vi "LLB - Header.vi"(7 "Msg Chain":string, 8 "error in (no error)":errorcluster {"code" format="Error %.0f"}, 10 "LLBs":refnum<class "LLB Documentation.lvclass">[](array[class]), 11 "VIDoc Printer - Confluence In":refnum<class "VIDoc Printer - Confluence.lvclass">) -> (0 "error out":errorcluster {"code" format="Error %.0f"}, 3 "VIDoc Printer - Confluence Out":refnum<class "VIDoc Printer - Confluence.lvclass">)   [LabVIEW 2023, in "VIDoc Printer - Confluence.lvlib" / "VIDoc Printer - Confluence.lvclass"]
uses:
  VIDoc Printer - Confluence.lvclass
  C:/projects/DMC/Tooling/Git-Action-Service/Source/Documentation Generation/Printers/Printer/VIDoc Printer.lvclass
  Parsing/LLB Documentation/LLB Documentation.lvclass
  Confluence Formatting/Types/Format Combo Box.ctl
  Parsing/LLB Documentation/LLB Documentation.lvclass/LLB Documentation.ctl
  Parsing/LLB Documentation/Get Name.vi
  VIDoc Printer - Confluence.lvclass/VIDoc Printer - Confluence.ctl
  Printer/VIDoc Printer.lvclass
  UI Interaction/UI Interaction.lvclass
  Confluence Formatting/Confluence Formatting.lvlib
  C:/projects/DMC/Tooling/Git-Action-Service/Source/Documentation Generation/Printers/Confluence Printer/VIDoc Printer - Confluence.lvclass
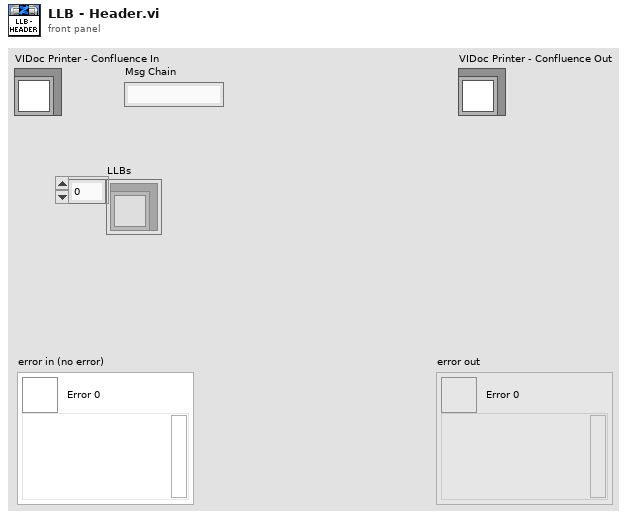
[diagram p1: front panel]
types:
  T1 = typedef "Confluence Formatting.lvlib/Format Combo Box.ctl" = string
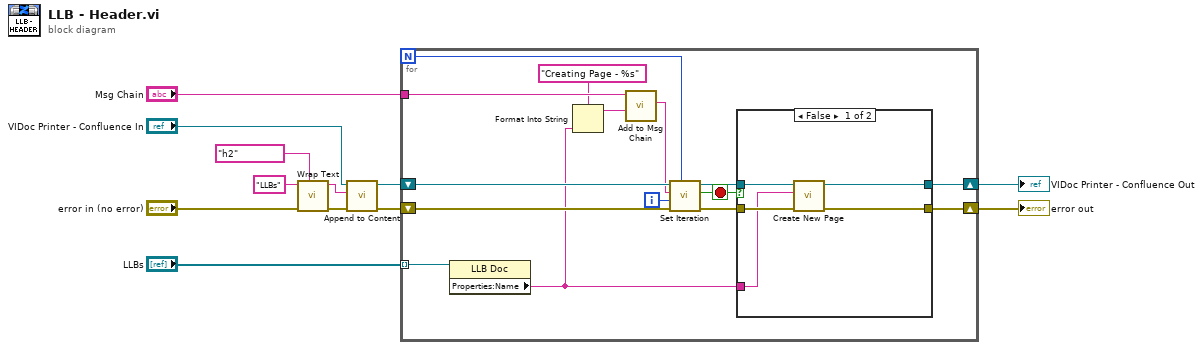
[diagram p0: block diagram]
diagram:
  n1 = call "Wrap Text.vi"("Formatting"=T1 "h2", "Error in"="error in (no error)", "String"="LLBs") -> ("Error out"=w11:errorcluster, "Wrapped String"=w10:string)  [unwired: 7 in]
  n2 = call "Append to Content.vi"("error in (no error)"=w11, "Content"=w10, "VIDoc Printer - Confluence In"="VIDoc Printer - Confluence In") -> ("error out"=w8:errorcluster, "VIDoc Printer - Confluence Out"=w7:refnum<class "VIDoc Printer - Confluence.lvclass">)  [unwired: 7 in]
  n3 = for {
    N -> [w20]
    shift-right: [w26] -> w4
    shift-left: w7 -> [w24]
    shift-right: [w27] -> w5
    shift-left: w8 -> [w23]
    tunnel: "LLBs" -> [w25] mode=indexing
    tunnel: "Msg Chain" -> [w18]
    i -> [w19]
    stop <- w13 stop-if-true
    n4 = property class="LLB Doc"(reference=w25) -> ("Properties:Name"=w14:string)  [unwired: 1 in, 2 out]
    n5 = Format Into String(format string="Creating Page - %s", w14) -> (resulting string=w16:string)  [unwired: 2 in, 1 out]
    n6 = call "Add to Msg Chain.vi"("New"=w16, "Msg Chain in"=w18) -> ("Msg Chain out"=w15:string)  [unwired: 9 in]
    n7 = call "Set Iteration.vi"("Progress Max"=w20, "error in (no error)"=w23, "Progress Value"=w19, "Message (No Message Update)"=w15, "VIDoc Printer In"=w24) -> ("error out"=w21:errorcluster, "Abort?"=w13:bool, "VIDoc Printer Out"=w22:refnum<class "VIDoc Printer - Confluence.lvclass">)  [unwired: 4 in]
    n8 = case shown="False" w13 {
      tunnel: [w30 w34] -> w27
      tunnel: [w29 w33] -> w26
      tunnel: w22 -> [w32 w33]
      tunnel: w21 -> [w31 w34]
      tunnel: w14 -> [w28 _]
      frame False {
        n9 = call "Create New Page.vi"("error in (no error)"=w31, "Name"=w28, "VIDoc Printer - Confluence In"=w32) -> ("error out"=w30:errorcluster, "VIDoc Printer - Confluence Out"=w29:refnum<class "VIDoc Printer - Confluence.lvclass">)  [unwired: 5 in, 2 out]
      }
      frame True {
      }
    }
  }
  "error out" <- w5
  "VIDoc Printer - Confluence Out" <- w4
